vi "同时终止两个循环.vi"() -> ()   [LabVIEW 2010]
uses:
  <vilib>/measure/NI_MABase.lvlib
panel:
  in  "停止":bool
  out "波形2":waveform(dbl)(graph)
  out "波形1":waveform(dbl)(graph)
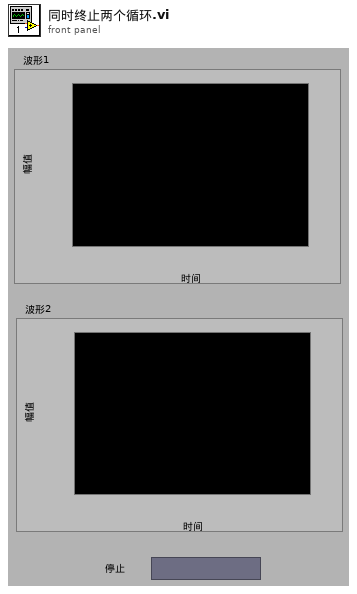
[diagram p1: front panel]
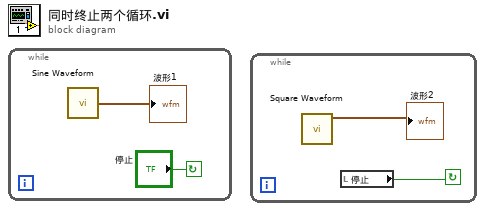
[diagram p0: block diagram]
diagram:
  n1 = while {
    stop <- "停止" continue-if-true
    n2 = call <vilib>:"Sine Waveform.vi"() -> ("signal out"=→"波形1":waveform(dbl))  [unwired: 10 in, 1 out]
  }
  n3 = while {
    stop <- w3 continue-if-true
    n4 = call <vilib>:"Square Waveform.vi"() -> ("signal out"=→"波形2":waveform(dbl))  [unwired: 10 in, 1 out]
    n5 = local read "停止"() -> (w3:bool)
  }
